vi "Time Acquisition Loop.vi"(0 "shared variable ref":refnum<k21> caption="共享变量引用", 3 "error in (no error)":errorcluster caption="错误输入（无错误）") -> (7 "Timestamp":timestamp caption="时间标识", 8 "Scan Engine Time":i64 caption="扫描引擎时间", 10 "error out":errorcluster caption="错误输出")   [LabVIEW 2015]
uses:
  <vilib>/Platform/TimedLoop/XDataNode/timing_clust.ctl
  <vilib>/Platform/TimedLoop/XDataNode/nitl_modes.ctl
  <vilib>/Platform/TimedLoop/XDataNode/wakeup.ctl
  <vilib>/Platform/TimedLoop/XDataNode/loadnilvce.vi
  Globals/Global - Configuration Options.vi
  <vilib>/Platform/TimedLoop/XDataNode/XDataNode.xnode
  <vilib>/Platform/TimedLoop/XDataNode/XDNodeRunTimeDep.lvlib
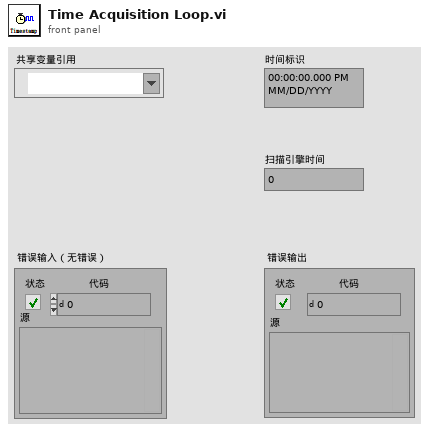
[diagram p1: front panel]
types:
  T1 = typedef "XDNodeRunTimeDep.lvlib/timing_clust.ctl" = cluster{"Expected End [f-1]":u64, "Actual End [f-1]":u64, "Finished Late? [f-1]":bool, "Expected End [i-1]":u64, "Actual End [i-1]":u64, "Finished Late? [i-1]":bool, "Expected Start [i]":u64, "Actual Start [i]":u64, "Expected Start [f]":u64, "Actual Start [f]":u64, "Source Name":string, "Structure Name":string, "Period":i64, "Deadline":i64, "Offset":i64, "Start":i64, "Priority":i32, "Timeout":i32, "Mode":T2, "Wakeup Reason":T3, "Error":errorcluster, "Source Type":string, "Secondary Source Type":string, "Global End Time":u64, "Global Start Time":u64, "Frame Duration":u64, "Iteration Duration":u64, "Assigned CPU":i32, "I/O Scan Engine Mode":u32}
  T2 = typedef "XDNodeRunTimeDep.lvlib/nitl_modes.ctl" = enum32{"No Change", "Process missed periods, maintain original phase", "Discard missed periods, maintain original phase", "Process missed periods, ignore original phase", "Discard missed periods, ignore original phase"}
  T3 = typedef "XDNodeRunTimeDep.lvlib/wakeup.ctl" = enum32{"Normal", "Aborted", "Asynchronous wakeup", "Timing source error", "Timed loop error", "Timeout"}
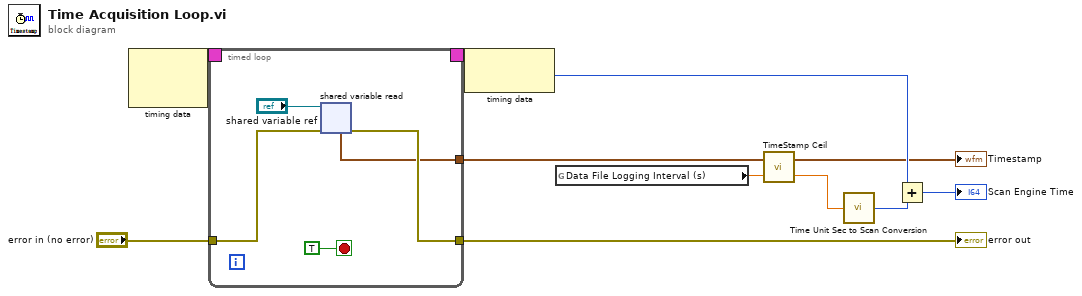
[diagram p0: block diagram]
diagram:
  n1 = node-c288() -> (w11:T1)  [unwired: 2 in]
  n2 = timed-loop {
    timing: w11 -> [_]
    timing-out: [_] -> w10
    tunnel: "error in (no error)" -> [w16]
    tunnel: [w13] -> w6
    tunnel: [w14] -> w1
    stop <- TRUE stop-if-true
    n3 = shared-variable-read("shared variable ref", w16) -> (w14:errorcluster, w13:timestamp)  [unwired: 2 out]
  }
  "error out" <- w1
  n4 = node-c288(w10) -> (w8:i64)
  n5 = global read "Global - Configuration Options.vi" "Data File Logging Interval (s)"() -> (w5:dbl)
  n6 = call "TimeStamp Ceil.vi"("base (s)"=w5, "timestamp input"=w6) -> ("time diff (s)"=w2:dbl, "timestamp output"=→"Timestamp":timestamp)
  n7 = call "Time Unit Sec to Scan Conversion.vi"("time duration (s)"=w2) -> ("time duration (scan)"=w3:i64)
  n8 = Add(x=w8, y=w3) -> (x+y=→"Scan Engine Time":i64)
